vi "channeldata_nodata.vi"() -> ()   [LabVIEW 2019]
panel:
  out "Error Out":errorcluster
  in  "TDMS File":path=path "C:/Python/projects/nitdms/tests/tdms_files/channeldata_nodata.tdms"
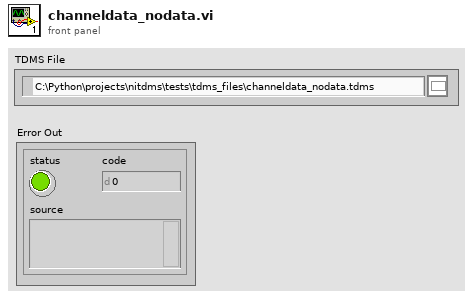
[diagram p1: front panel]
types:
  T1 = enum16{"open", "open or create", "create or replace", "create", "open (read-only)"}
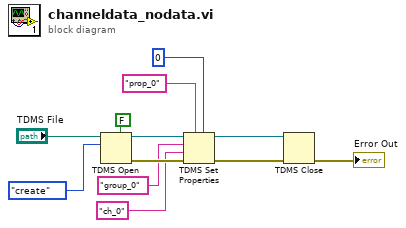
[diagram p0: block diagram]
diagram:
  n1 = TDMS Open(5:FALSE ("create index file? (T)"), 10:T1."create" ("operation (0:open)"), 11:"TDMS File") -> (0:w8:errorcluster, 3:w5:refnum<k34>)  [unwired: 4 in]
  n2 = TDMS Set Properties(5:0, 7:"prop_0", 8:w8, 9:"ch_0", 10:"group_0", 11:w5) -> (0:w7:errorcluster, 3:w6:refnum<k34>)  [unwired: 2 out]
  n3 = TDMS Close(8:w7, 11:w6) -> (0:→"Error Out":errorcluster)  [unwired: 1 out]
